vi "NonLinearMixer.vi"() -> ()   [LabVIEW 2009]
uses:
  <vilib>/Analysis/4window.llb/windowTd.ctl
  <vilib>/measure/maspectr.llb/FFT Power Spectrum for 1 Chan.vi
  <vilib>/measure/NI_MAPro.lvlib
  <vilib>/Analysis/NI_AALPro.lvlib
panel:
  in  "Tab Control":enum32{"Distortion Input", "Mixer Output"}(tab)=enum."Mixer Output"
  out "Post Distortion RF input":cluster{"f0":dbl, "df":dbl, "magnitude":dbl[]}(graph)={"f0"=0.0, "df"=100000.00000000001, "magnitude"=array[24563 elements]}
  out "Post Distortion LO input":cluster{"f0":dbl, "df":dbl, "magnitude":dbl[]}(graph)={"f0"=0.0, "df"=100000.00000000001, "magnitude"=array[24563 elements]}
  out "Ideal  (Linear) Mixer output":cluster{"f0":dbl, "df":dbl, "magnitude":dbl[]}(graph)={"f0"=0.0, "df"=100000.00000000001, "magnitude"=array[24563 elements]}
  out "Distorted Mixer output with LO->IF and RF->IF Leakage":cluster{"f0":dbl, "df":dbl, "magnitude":dbl[]}(graph)={"f0"=0.0, "df"=100000.00000000001, "magnitude"=array[24563 elements]}
  in  "Show Image Band":bool
  in  "RF -> IF Leakage (in dBc)":dbl=-30.0
  in  "LO -> IF Leakage (in dBc)":dbl=-30.0
  out "LO Frequency (Hz)":dbl=960000000.0 format="%#_6p"
  out "RF input":cluster{"f0":dbl, "df":dbl, "magnitude":dbl[]}(graph)={"f0"=0.0, "df"=100000.00000000001, "magnitude"=array[24563 elements]}
  in  "RF Gain Terms (first gain term applied to linear part)":dbl[](array[numeric])=[1.0, 0.001, 0.0, 0.0, 0.0] format="%.2p"
  in  "LO Gain Terms  (first gain term applied to linear part)":dbl[](array[numeric])=[1.0, 0.001, 0.0, 0.0, 0.0] format="%.2p"
  in  "Tuning":bool caption="Low Side / High Side tuning"
  in  "Duration (Seconds)":dbl=1e-05
  in  "RF Passband Bandwidth (Hz)":dbl=10000000.0 format="%#_6p"
  in  "Intermediate Frequency":dbl=40000000.0 format="%#_6p"
  in  "RF Carrier Frequency":dbl=1000000000.0 format="%#_6p"
  in  "Integer Degree of Nonlinearity (LO)":i32=1
  in  "Integer Degree of Nonlinearity (RF)":i32=1
  # "The image band is occupied by the 'pointy' spectra"
  # "*For more information on each a control,\nPlease see the description for that control"
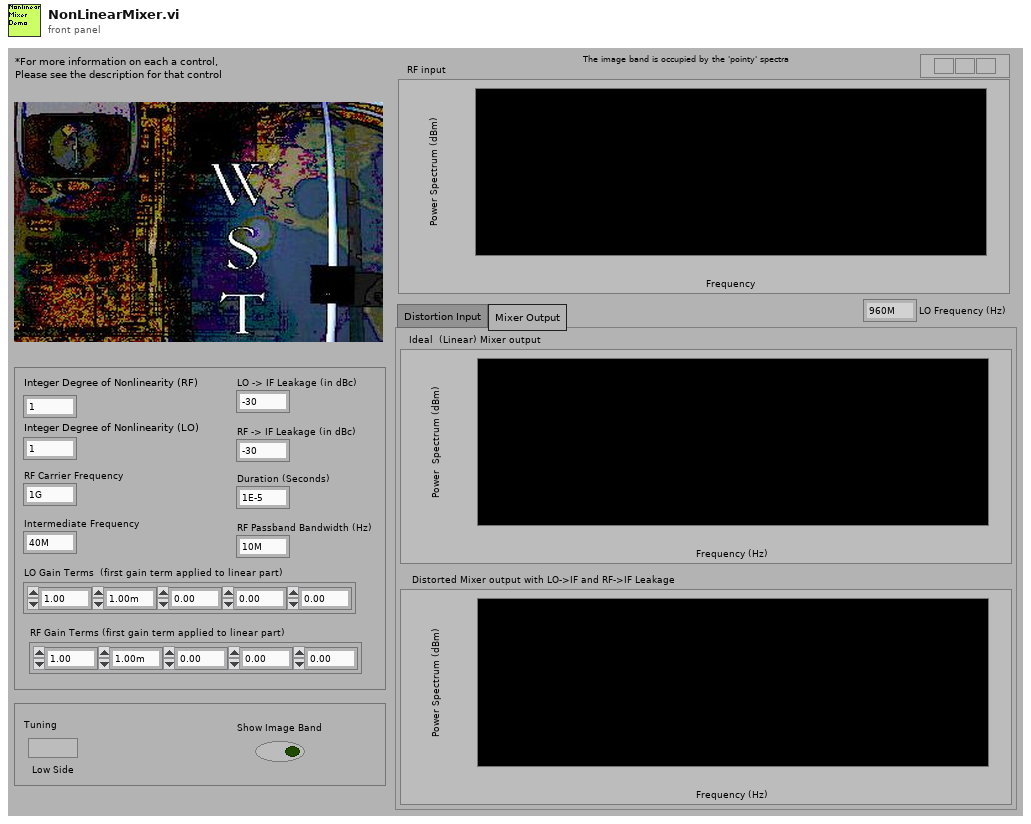
[diagram p1: front panel]
types:
  T1 = typedef "NI_AALPro.lvlib/windowTd.ctl" = u32
  T2 = cluster{" Sampling Frequency":dbl, "Number of Samples":dbl}
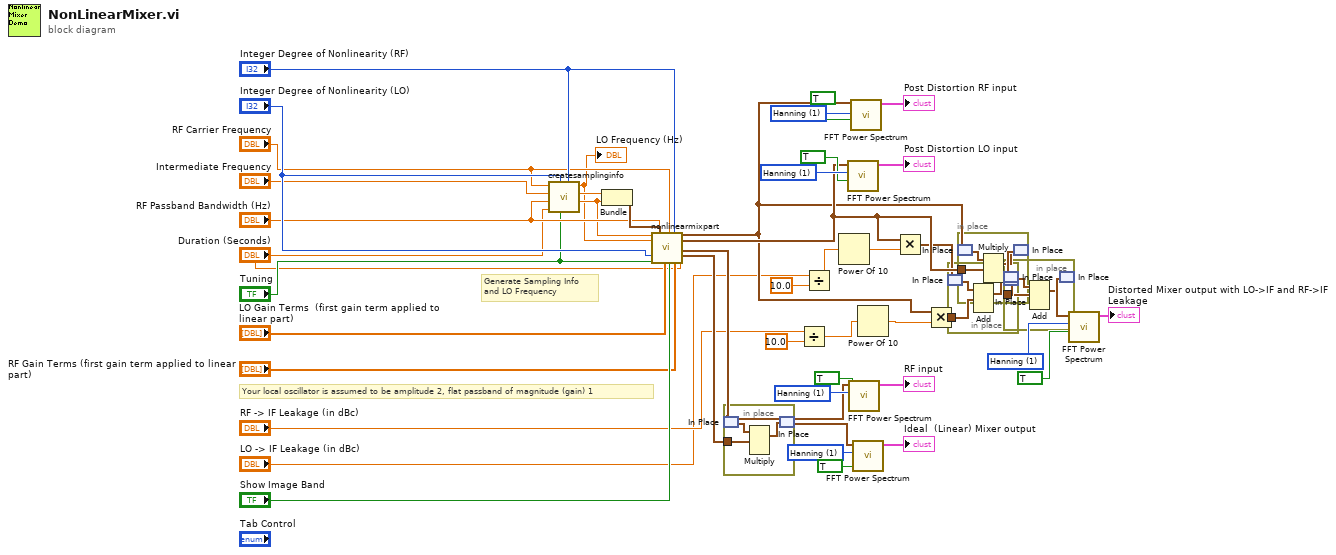
[diagram p0: block diagram]
diagram:
  w32 = T1 1 items=["Rectangle"=0, "Hanning"=1, "Hamming"=2, "Blackman-Harris"=3, "Exact Blackman"=4, "Blackman"=5, "Flat Top"=6, "4 Term B-Harris "=7, "7 Term B-Harris"=8, "Low Sidelobe"=9, "Blackman Nuttall"=11, "Triangle"=30, "Kaiser"=60, "Dolph-Chebyshev"=61, "Gaussian"=62] ("window")
  w35 = T1 1 items=["Rectangle"=0, "Hanning"=1, "Hamming"=2, "Blackman-Harris"=3, "Exact Blackman"=4, "Blackman"=5, "Flat Top"=6, "4 Term B-Harris "=7, "7 Term B-Harris"=8, "Low Sidelobe"=9, "Blackman Nuttall"=11, "Triangle"=30, "Kaiser"=60, "Dolph-Chebyshev"=61, "Gaussian"=62] ("window")
  w39 = T1 1 items=["Rectangle"=0, "Hanning"=1, "Hamming"=2, "Blackman-Harris"=3, "Exact Blackman"=4, "Blackman"=5, "Flat Top"=6, "4 Term B-Harris "=7, "7 Term B-Harris"=8, "Low Sidelobe"=9, "Blackman Nuttall"=11, "Triangle"=30, "Kaiser"=60, "Dolph-Chebyshev"=61, "Gaussian"=62] ("window")
  w44 = T1 1 items=["Rectangle"=0, "Hanning"=1, "Hamming"=2, "Blackman-Harris"=3, "Exact Blackman"=4, "Blackman"=5, "Flat Top"=6, "4 Term B-Harris "=7, "7 Term B-Harris"=8, "Low Sidelobe"=9, "Blackman Nuttall"=11, "Triangle"=30, "Kaiser"=60, "Dolph-Chebyshev"=61, "Gaussian"=62] ("window")
  w45 = T1 1 items=["Rectangle"=0, "Hanning"=1, "Hamming"=2, "Blackman-Harris"=3, "Exact Blackman"=4, "Blackman"=5, "Flat Top"=6, "4 Term B-Harris "=7, "7 Term B-Harris"=8, "Low Sidelobe"=9, "Blackman Nuttall"=11, "Triangle"=30, "Kaiser"=60, "Dolph-Chebyshev"=61, "Gaussian"=62] ("window")
  # "Your local oscillator is assumed to be amplitude 2, flat passband of magnitude (gain) 1"
  # "Generate Sampling Info\nand LO Frequency"
  n1 = call "createsamplinginfo.vi"("Integer Degree of Nonlinearity (RF) (N) ( y(t) = x^1(t) + ...  + x^N(t) )"="Integer Degree of Nonlinearity (RF)", "Low Side / High Side tuning"="Tuning", "Integer Degree of Nonlinearity (LO) (N) ( y(t) = x^1(t) + ...  + x^N(t) )"="Integer Degree of Nonlinearity (LO)", "Duration (Seconds)"="Duration (Seconds)", "RF Passband Bandwidth (Hz)"="RF Passband Bandwidth (Hz)", "Intermediate Frequency"="Intermediate Frequency", "RF Carrier Frequency"="RF Carrier Frequency") -> ("Number of Samples"=w2:dbl, "Sampling Frequency"=w3:dbl, "LO Frequency"=w1:dbl)  [unwired: 2 in]
  "LO Frequency (Hz)" <- w1
  n2 = Bundle("Sampling Frequency"=w3, "Number of Samples"=w2) -> (w47:T2)  [unwired: 1 in]
  n3 = call "nonlinearmixpart.vi"("Number of Samples"=w2, "LO Frequency"=w1, "Integer Degree of Nonlinearity (LO) (N) ( y(t) = x^1(t) + ...  + x^N(t) )"="Integer Degree of Nonlinearity (LO)", "Low Side / High Side"="Tuning", "Sampling Info"=w47, "RF Passband Bandwidth (Hz)"="RF Passband Bandwidth (Hz)", "LO Gain Terms  (first gain term applied to linear part)"="LO Gain Terms  (first gain term applied to linear part)", "RF Carrier Frequency"="RF Carrier Frequency", "Show Image Band"="Show Image Band", "Integer Degree of Nonlinearity (RF) (N) ( y(t) = x^1(t) + ...  + x^N(t) )"="Integer Degree of Nonlinearity (RF)", "RF Gain Terms (first gain term applied to linear part)"="RF Gain Terms (first gain term applied to linear part)", "Duration (Seconds)"="Duration (Seconds)") -> ("Post Distortion Passband Waveform"=w22:waveform(dbl), "Post-distortion Local Oscillator Waveform"=w27:waveform(dbl), "Pre-distortion passband waveform"=w37:waveform(dbl), "Pre-distortion Local Oscillator Waveform"=w46:waveform(dbl))  [unwired: 4 in]
  n4 = in-place {
    in-place-border: w46 -> [w50]
    n5 = in-place-match #1(w37) -> (w49:waveform(dbl))
    n6 = Multiply(1:w50, 2:w49) -> (0:w48:waveform(dbl))  [unwired: 1 in, 1 out]
    n7 = in-place-match #1(w48) -> (w15:waveform(dbl))
  }
  n8 = Divide(x="RF -> IF Leakage (in dBc)", y=10.0) -> (x/y=w24:dbl)
  n9 = Divide(x="LO -> IF Leakage (in dBc)", y=10.0) -> (x/y=w28:dbl)
  n10 = Power Of 10(x=w28) -> (10^x=w26:dbl)
  n11 = call-poly <vilib>:"FFT Power Spectrum.vi"("dB On (F)"=TRUE, "window"=w35, "time signal"=w27) -> ("power spectrum"=→"Post Distortion LO input":cluster{"f0":dbl, "df":dbl, "magnitude":dbl[]})  [unwired: 5 in, 3 out]
  n12 = call-poly <vilib>:"FFT Power Spectrum.vi"("dB On (F)"=TRUE, "window"=w39, "time signal"=w37) -> ("power spectrum"=→"RF input":cluster{"f0":dbl, "df":dbl, "magnitude":dbl[]})  [unwired: 5 in, 3 out]
  n13 = call-poly <vilib>:"FFT Power Spectrum.vi"("dB On (F)"=TRUE, "window"=w32, "time signal"=w22) -> ("power spectrum"=→"Post Distortion RF input":cluster{"f0":dbl, "df":dbl, "magnitude":dbl[]})  [unwired: 5 in, 3 out]
  n14 = call-poly <vilib>:"FFT Power Spectrum.vi"("dB On (F)"=TRUE, "window"=w45, "time signal"=w15) -> ("power spectrum"=→"Ideal  (Linear) Mixer output":cluster{"f0":dbl, "df":dbl, "magnitude":dbl[]})  [unwired: 5 in, 3 out]
  n15 = Power Of 10(x=w24) -> (10^x=w23:dbl)
  n16 = Multiply(x=w27, y=w26) -> (x*y=w21:waveform(dbl))
  n17 = Multiply(x=w22, y=w23) -> (x*y=w20:waveform(dbl))
  n18 = in-place {
    in-place-border: w20 -> [w52]
    n19 = in-place-match #2(w21) -> (w53:waveform(dbl))
    n20 = Add(1:w52, 2:w53) -> (0:w51:waveform(dbl))  [unwired: 1 in, 1 out]
    n21 = in-place-match #2(w51) -> (w18:waveform(dbl))
  }
  n22 = in-place {
    in-place-border: w27 -> [w56]
    n23 = in-place-match #3(w22) -> (w55:waveform(dbl))
    n24 = Multiply(1:w56, 2:w55) -> (0:w54:waveform(dbl))  [unwired: 1 in, 1 out]
    n25 = in-place-match #3(w54) -> (w19:waveform(dbl))
  }
  n26 = in-place {
    in-place-border: w18 -> [w58]
    n27 = in-place-match #4(w19) -> (w59:waveform(dbl))
    n28 = Add(1:w58, 2:w59) -> (0:w57:waveform(dbl))  [unwired: 1 in, 1 out]
    n29 = in-place-match #4(w57) -> (w17:waveform(dbl))
  }
  n30 = call-poly <vilib>:"FFT Power Spectrum.vi"("dB On (F)"=TRUE, "window"=w44, "time signal"=w17) -> ("power spectrum"=→"Distorted Mixer output with LO->IF and RF->IF Leakage":cluster{"f0":dbl, "df":dbl, "magnitude":dbl[]})  [unwired: 5 in, 3 out]
